vi "timedependent_writing_and_waveform_chart.vi"() -> ()   [LabVIEW 2019]
panel:
  out "Waveform Chart":dbl[](graph)
  out "Döngü":i32
  in  "stop":bool
  out "sıcaklık1":dbl
  out "sıcaklık2":dbl
  out "sıcaklık3":dbl
  out "String":string
  in  "file path":path
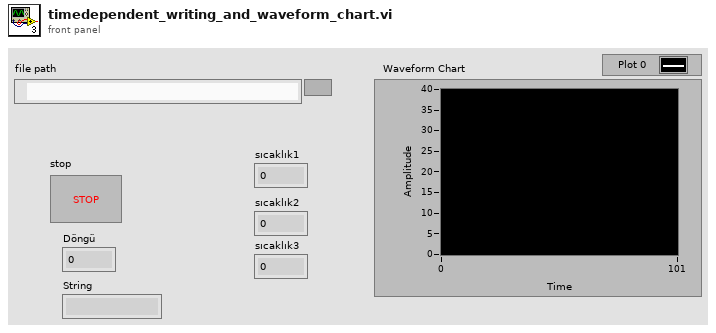
[diagram p1: front panel]
types:
  T1 = enum16{"open", "replace", "create", "open or create", "replace or create", "replace or create with confirmation"}
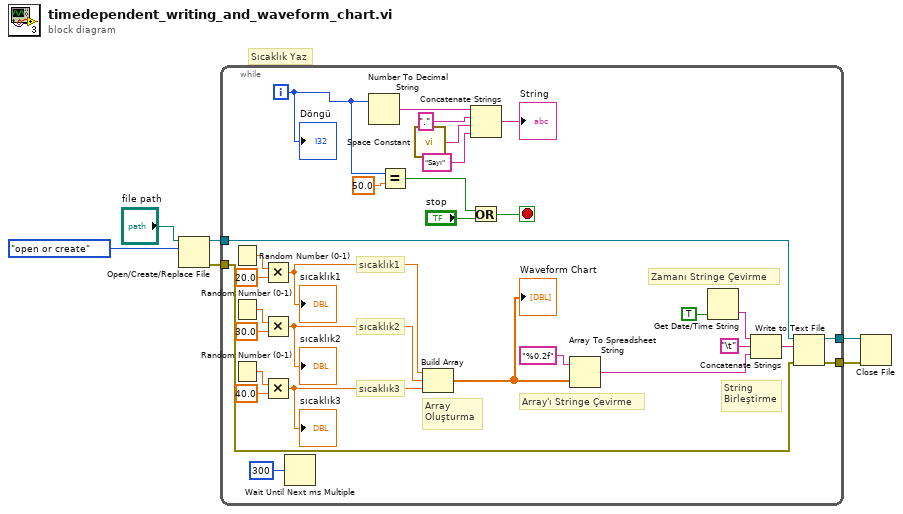
[diagram p0: block diagram]
diagram:
  # "Sıcaklık Yaz"
  n1 = Open/Create/Replace File(file path (use dialog)="file path", operation (0:open)=T1."open or create") -> (refnum out=w4:refnum<file>, error out=w1:errorcluster)  [unwired: 4 in, 1 out]
  n2 = while {
    tunnel: w4 -> [w37]
    tunnel: [w36] -> w3
    tunnel: [w35] -> w2
    tunnel: w1 -> [w34]
    i -> [w12]
    stop <- w23 stop-if-true
    # "String \nBirleştirme"
    # "Array'ı Stringe Çevirme"
    # "Zamanı Stringe Çevirme"
    # "Array \nOluşturma"
    # "sıcaklık3"
    # "sıcaklık2"
    # "sıcaklık1"
    n3 = Random Number (0-1)() -> (number: 0 to 1=w33:dbl)
    n4 = Random Number (0-1)() -> (number: 0 to 1=w21:dbl)
    n5 = Random Number (0-1)() -> (number: 0 to 1=w19:dbl)
    n6 = Multiply(x=w33, y=20.0) -> (x*y=w16:dbl)
    "sıcaklık1" <- w16
    n7 = Multiply(x=w21, y=30.0) -> (x*y=w15:dbl)
    "sıcaklık2" <- w15
    n8 = Multiply(x=w19, y=40.0) -> (x*y=w14:dbl)
    "sıcaklık3" <- w14
    n9 = Wait Until Next ms Multiple(millisecond multiple=u32 300) -> ()  [unwired: 1 out]
    n10 = Number To Decimal String(number=w12) -> (decimal integer string=w7:string)  [unwired: 1 in]
    n11 = Equal?(x=w12, y=50.0) -> (x = y?=w22:bool)
    n12 = call <vilib>:"Space Constant.vi"() -> ("String"=w10:string)
    n13 = Build Array(w16, w15, w14) -> (w30:dbl[])
    "Waveform Chart" <- w30
    n14 = Concatenate Strings(w7, "." ("string"), w10, "Sayı" ("string")) -> (→"String":string)
    n15 = Or(x=w22, y="stop") -> (x .or. y?=w23:bool)
    n16 = Array To Spreadsheet String(array=w30, 3:"%0.2f" ("format string")) -> (spreadsheet string=w27:string)  [unwired: 1 in]
    n17 = Get Date/Time String(want seconds? (F)=TRUE) -> (time string=w29:string)  [unwired: 2 in, 1 out]
    n18 = Concatenate Strings(w29, "\t", w27) -> (w13:string)
    n19 = Write to Text File(file (use dialog)=w37, text=w13, error in=w34) -> (refnum out=w36:refnum<file>, error out=w35:errorcluster)  [unwired: 1 in, 1 out]
    "Döngü" <- w12
  }
  n20 = Close File(refnum=w3, error in=w2) -> ()  [unwired: 2 out]
